vi "PH_Beckhoff_PP_PU.set further GUI Objects.vi"(0 "VI in":refnum<vi>, 2 "Refs HV Meas":refnum<vi>[](array[refnum]), 3 "Refs Voltage":refnum<vi>[](array[refnum]), 5 "error in (no error)":errorcluster) -> (14 "VI out":refnum<vi>, 15 "Type PSU 1":T1, 16 "Type PSU 2":T1, 17 "PU Rack Type":T2, 19 "error out":errorcluster)   [LabVIEW 2014, in "PH_Beckhoff_PP_PU.lvlib"]
uses:
  PH_Beckhoff_PP_PU.lvlib
  PH_Beckhoff_PP_PU.PU Rack Type.ctl
  PH_Basics/PH_PP_Common/PH_PP_Common.PSU Type.ctl
  PH_Beckhoff_PP_PU.HV Meas Tags.ctl
  PH_Basics/PH_PP_Common/PH_PP_Common.PSU Tags.ctl
  PH_Basics/PH_PP_Common/PH_PP_Common.lvlib
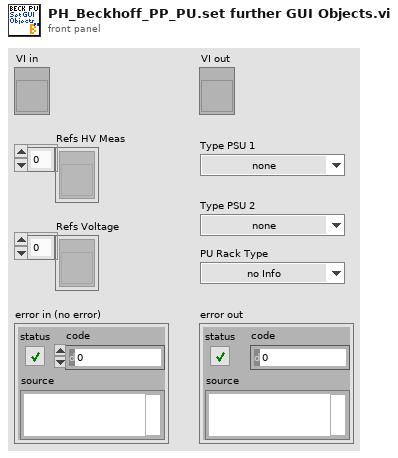
[diagram p1: front panel]
types:
  T1 = typedef "PH_PP_Common.lvlib/PH_PP_Common.PSU Type.ctl" = enum16{"none", "Maxwell Standard", "DEL", "Maxwell ALE", "Continuum 601k"}
  T2 = typedef "PH_Beckhoff_PP_PU.lvlib/PH_Beckhoff_PP_PU.PU Rack Type.ctl" = enum16{"no Info", "PA 19mm", "PA 45mm", "MA PU 1 and 2", "MA PU 3 and 4", "MA PU 5 and 6", "MA FR and PILC"}
  T3 = typedef "PH_PP_Common.lvlib/PH_PP_Common.PSU Tags.ctl" = enum16{"voltage-indicator", "peak-detect", "current", "voltage", "inihibit-indicator", "end-of-charge", "HV-on-indicator", "overtemperature", "interlock-indicator", "load-fault", "sum-fault", "HV-off-indicator", "DC-ok", "inhibit", "HV-on", "interlock", "reset", "Status", "Limits"}
  T4 = typedef "PH_Beckhoff_PP_PU.lvlib/PH_Beckhoff_PP_PU.HV Meas Tags.ctl" = enum16{"voltage-raw", "voltage"}
  T5 = typedef "PH_PP_Common.lvlib/PH_PP_Common.PUs.ctl" = enum16{"no Info", "PA-19mm-1", "PA-19mm-2", "PA-45mm-PILC", "PA-45mm-MAIN", "MA-PU-1", "MA-PU-2", "MA-PU-3", "MA-PU-4", "MA-PU-5", "MA-PU-6", "MA-FR", "MA-PILC", "PA-45mm-DP"}
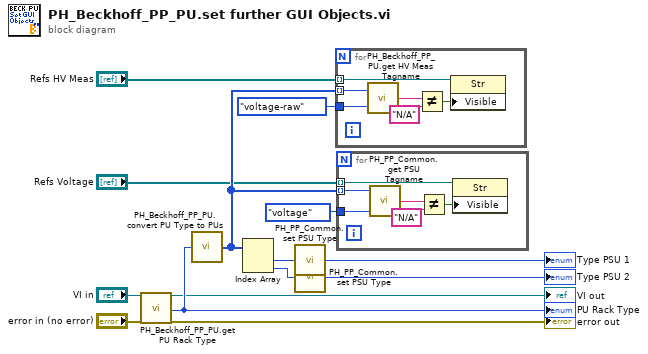
[diagram p0: block diagram]
diagram:
  n1 = call "PH_Beckhoff_PP_PU.get PU Rack Type.vi"("VI in"="VI in", "error in (no error)"="error in (no error)") -> ("VI out"=→"VI out":refnum<vi>, "PU Rack Type"=w12:T2, "error out"=→"error out":errorcluster)  [unwired: 15 in]
  "PU Rack Type" <- w12
  n2 = call "PH_Beckhoff_PP_PU.convert PU Type to PUs.vi"("PU Type"=w12) -> ("PUs"=w6:T5[])
  n3 = Index Array(array=w6) -> (element #1=w9:T5, element #2=w8:T5)  [unwired: 2 in]
  n4 = call "PH_PP_Common.set PSU Type.vi"("PU"=w9) -> ("PSU Type"=→"Type PSU 1":T1)
  n5 = call "PH_PP_Common.set PSU Type.vi"("PU"=w8) -> ("PSU Type"=→"Type PSU 2":T1)
  n6 = for {
    tunnel: w6 -> [w20] mode=indexing
    tunnel: PH_Beckhoff_PP_PU.HV_Meas_Tags."voltage-raw" ("HV Meas Tag") -> [w19]
    tunnel: "Refs HV Meas" -> [w16] mode=indexing
    n7 = call "PH_Beckhoff_PP_PU.get HV Meas Tagname.vi"("HV Meas Tag"=w19, "PU"=w20) -> ("HV Meas Tagname"=w18:string)
    n8 = Not Equal?(x=w18, y="N/A") -> (x != y?=w15:bool)
    n9 = property class="Str"(reference=w16, "Visible"=w15) -> ()  [unwired: 1 in, 2 out]
  }
  n10 = for {
    tunnel: w6 -> [w26] mode=indexing
    tunnel: "Refs Voltage" -> [w23] mode=indexing
    tunnel: PH_PP_Common.PSU_Tags."voltage" ("PSU Tag") -> [w21]
    n11 = call "PH_PP_Common.get PSU Tagname.vi"("PSU Tag"=w21, "PU"=w26) -> ("PSU Tagname"=w25:string)  [unwired: 1 in]
    n12 = Not Equal?(x=w25, y="N/A") -> (x != y?=w22:bool)
    n13 = property class="Str"(reference=w23, "Visible"=w22) -> ()  [unwired: 1 in, 2 out]
  }
